vi "ZCAN_OpenDevice.vi"(8 "error in (no error)":errorcluster caption="错误输入（无错误）", 9 "reserved":u32, 10 "device_index":u32, 11 "device_type":u32) -> (0 "error out":errorcluster caption="错误输出", 2 "DEVICE_HANDLE":u64)   [LabVIEW 2018, in "zlgcan.lvlib"]
doc: "该函数用于打开设备，一个设备只能被打开一次，返回值为设备句柄。\n注意：关闭程序前要调用ZCAN_CloseDevice释放设备句柄，否则第二次无法打开；\n\n如忘记释放句柄，需要关闭整个LabVIEW程序，CAN卡重新插拔。"
uses:
  zlgcan.lvlib
  bin/ControlCANFD.dll
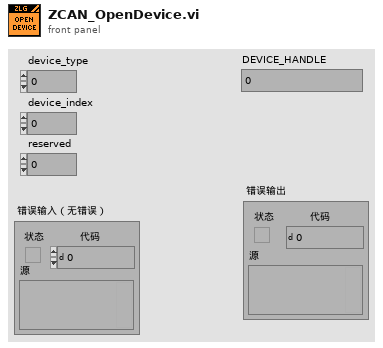
[diagram p1: front panel]
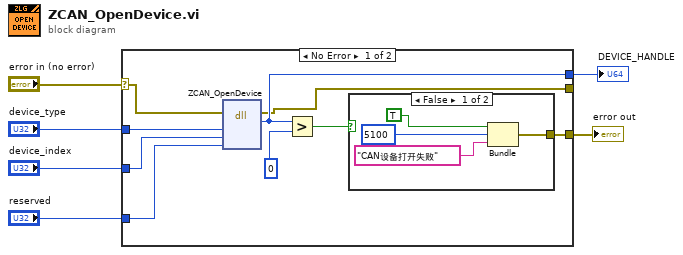
[diagram p0: block diagram]
diagram:
  n1 = case shown="No Error" "error in (no error)" {
    selector: "error in (no error)" -> [w11 w20]
    tunnel: [w9 w20] -> w5
    tunnel: "device_type" -> [w15 _]
    tunnel: "device_index" -> [w14 _]
    tunnel: "reserved" -> [w13 _]
    tunnel: [w8 _] -> w1
    tunnel: [w7 _] -> _
    frame No Error {
      n2 = dll-call lib="C:/Users/ttc52/Desktop/DHC FD LV2018/LABIVIEW CANFD Tool_V1.2.4_20220724/bin/ControlCANFD.dll" fn="ZCAN_OpenDevice"(error in=w11, "device_type"=w15, "device_index"=w14, "reserved"=w13) -> (error out=w7:errorcluster, "DEVICE_HANDLE"=w8:u64)  [unwired: 5 in, 1 out]
      n3 = Greater?(x=w8, y=u32 0) -> (0:w10:bool)
      n4 = case shown="False" w10 {
        tunnel: [w18 _] -> w9
        frame False {
          n5 = Bundle("status"=TRUE, "code"=5100, "消息"="CAN设备打开失败") -> (w18:cluster{"status":bool, "code":i32, "消息":string})  [unwired: 1 in]
        }
        frame True {
        }
      }
    }
    frame Error {
    }
  }
  "error out" <- w5
  "DEVICE_HANDLE" <- w1
